vi "Increment I32 by Reference.vi"(0 "error in":errorcluster, 2 "step size (1)":i32=1 step=1, 3 "dignum refnum":refnum<vi>, 4 "enable (T)":bool=TRUE) -> (7 "error out":errorcluster, 9 "value":i32, 10 "dignum refnum dup":refnum<vi>)   [LabVIEW 2010]
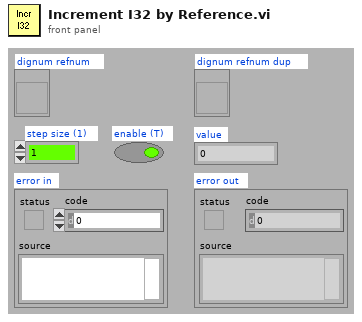
[diagram p1: front panel]
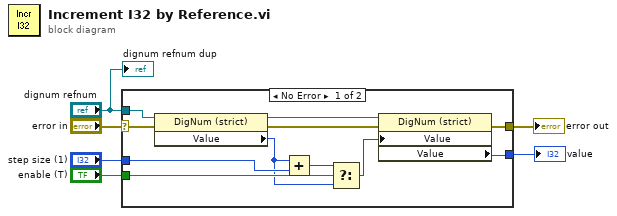
[diagram p0: block diagram]
diagram:
  n1 = case shown="No Error" "error in" {
    selector: "error in" -> [w15 w17]
    tunnel: [w12 w17] -> w5
    tunnel: "dignum refnum" -> [w16 _]
    tunnel: [w10 _] -> w3
    tunnel: "enable (T)" -> [w11 _]
    tunnel: "step size (1)" -> [w8 _]
    frame No Error {
      n2 = property class="DigNum (strict)"(reference=w16, error in=w15) -> (reference out=w14:refnum<vi>, error out=w13:errorcluster, "Value"=w7:i32)
      n3 = Add(x=w7, y=w8) -> (x+y=w9:i32)
      n4 = Select(t=w9, s=w11, f=w7) -> (s? t:f=w10:i32)
      n5 = property class="DigNum (strict)" props=["Value", "Value"](reference=w14, error in=w13, "Value"=w10) -> (error out=w12:errorcluster)  [unwired: 2 out]
    }
    frame Error {
    }
  }
  "error out" <- w5
  "value" <- w3
  "dignum refnum dup" <- "dignum refnum"
